vi "Encoder_sub_VI.vi"(8 "error in (no error)":errorcluster, 11 "Encoder Input":T2) -> (0 "error out":errorcluster, 3 "Encoder Output":T2)   [LabVIEW 2017]
uses:
  <vilib>/myRIO/Common/Instrument Driver Framework/myRIO v1.0/Encoder/typedefs/Encoder Count Direction Enum.ctl
  <vilib>/myRIO/Common/Instrument Driver Framework/myRIO v1.0/Encoder/typedefs/Encoder Signal Mode.ctl
  <vilib>/myRIO/Instrument Drivers/Onboard IO/Encoder/typedefs/Encoder Reference.ctl
  <vilib>/myRIO/Common/Instrument Driver Framework/Utilities/typedefs/myRIO Generic Hardware Reference.ctl
  <vilib>/myRIO/Common/Instrument Driver Framework/Utilities/typedefs/Hardware Version Enum.ctl
  <vilib>/myRIO/Common/Instrument Driver Framework/Utilities/typedefs/myRIO v1.0 Reference.ctl
  <vilib>/myRIO/Common/Instrument Driver Framework/Utilities/typedefs/Generic FPGA Reference.ctl
  <vilib>/myRIO/Common/Instrument Driver Framework/myRIO v1.0/Encoder/typedefs/Encoder Channels Enum.ctl
  <vilib>/myRIO/Common/Instrument Driver Framework/myRIO v1.0/Encoder/typedefs/Encoder Configuration v1.0.ctl
  <vilib>/userdefined/High Color/nirio_resource_hc.ctl
  <vilib>/myRIO/Common/Instrument Driver Framework/Utilities/vis/Is FPGA Ref Available.vi
  <vilib>/myRIO/Common/Instrument Driver Framework/myRIO v1.0/Encoder/vis/myRIO v1.1 Open Encoder.vi
  <vilib>/myRIO/Instrument Drivers/Onboard IO/Encoder/vis/Read.vi
  <vilib>/myRIO/Common/Instrument Driver Framework/Utilities/vis/Validate Channels.vi
  <vilib>/myRIO/Common/Instrument Driver Framework/myRIO v1.0/Encoder/vis/myRIO v1.0 Reserve Encoder.vi
  <vilib>/myRIO/Common/Instrument Driver Framework/myRIO v1.0/Encoder/vis/myRIO v1.0 Build MUX Configuration Encoder.vi
  <vilib>/myRIO/Common/Instrument Driver Framework/myRIO v1.0/Resource Manager/vis/myRIO v1.0 Reserve Channel List.vi
  <vilib>/myRIO/Common/Instrument Driver Framework/myRIO v1.0/Resource Manager/vis/myRIO v1.0 Create Configuration List.vi
  <vilib>/myRIO/Common/Instrument Driver Framework/myRIO v1.0/Resource Manager/vis/myRIO v1.0 Reserve Channel.vi
  <vilib>/myRIO/Common/Instrument Driver Framework/myRIO v1.0/Resource Manager/vis/myRIO v1.0 Unreserve Channel.vi
  <vilib>/myRIO/Common/Instrument Driver Framework/myRIO v1.0/Resource Manager/vis/myRIO v1.0 Build Mutex Name.vi
  <vilib>/Utility/VariantDataType/GetNumericInfo.vi
  <vilib>/Utility/error.llb/Error Cluster From Error Code.vi
  <vilib>/myRIO/Common/Instrument Driver Framework/myRIO v1.0/myRIO v1.1 Open.vi
  <vilib>/myRIO/Common/Instrument Driver Framework/Utilities/vis/IO Manager.vi
  <vilib>/myRIO/Common/Instrument Driver Framework/Utilities/vis/Configuration Manager.vi
  <vilib>/myRIO/Common/Instrument Driver Framework/myRIO v1.0/Resource Manager/vis/myRIO v1.0 Configure IO.vi
  <vilib>/myRIO/Common/Instrument Driver Framework/myRIO v1.0/myRIO v1.0 Close.vi
  <vilib>/myRIO/Common/Instrument Driver Framework/myRIO v1.0/Encoder/vis/myRIO v1.0 Configure Encoder.vi
  <vilib>/myRIO/Common/Instrument Driver Framework/myRIO v1.0/Encoder/vis/myRIO v1.0 Read Encoder.vi
  <vilib>/myRIO/Express VI/Onboard IO/Encoder/Encoder Express VI.xnode
  <vilib>/myRIO/Instrument Drivers/Onboard IO/Encoder/vis/myRIO Encoder Open.xnode
  <vilib>/myRIO/Instrument Drivers/Onboard IO/Encoder/Encoder.lvlib
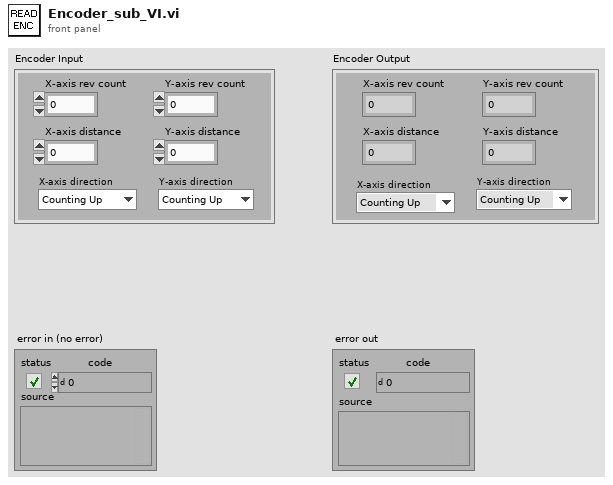
[diagram p1: front panel]
types:
  T1 = typedef "Encoder Count Direction Enum.ctl" = enum16{"Counting Up", "Counting Down"}
  T2 = cluster{"Y-axis rev count":dbl, "Y-axis distance":dbl, "X-axis rev count":dbl, "X-axis distance":dbl, "Y-axis direction":T1, "X-axis direction":T1}
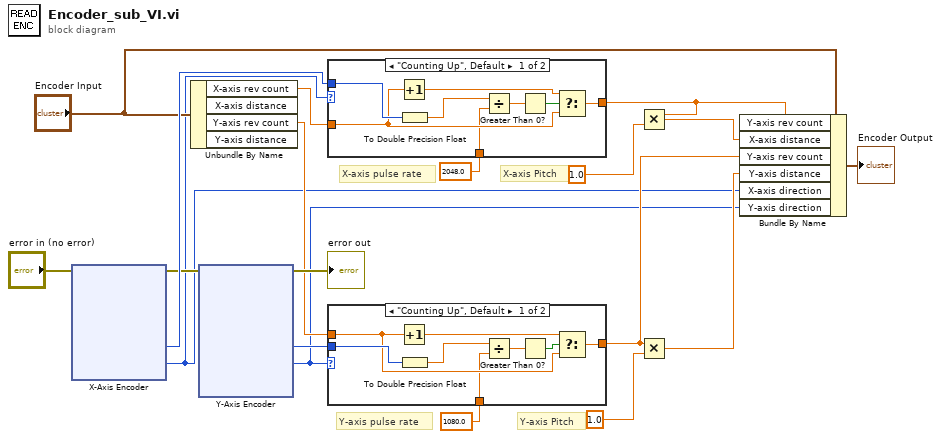
[diagram p0: block diagram]
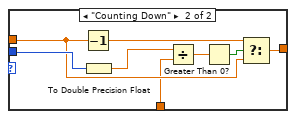
[diagram p2: hidden frame]
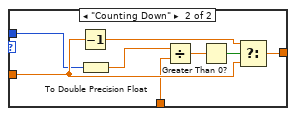
[diagram p3: hidden frame]
diagram:
  # "Y-axis pulse rate"
  # "X-axis pulse rate"
  # "Y-axis Pitch"
  # "X-axis Pitch"
  n1 = xnode "X-Axis Encoder"("error in (no error)"="error in (no error)") -> ("Counter Value"=w16:i32, "Counter Direction"=w2:T1, "error out"=w14:errorcluster)  [unwired: 1 in, 1 out]
  n2 = Unbundle By Name("Encoder Input") -> ("X-axis rev count"=w6:dbl, "Y-axis rev count"=w7:dbl)  [unwired: 2 out]
  n3 = xnode "Y-Axis Encoder"("error in (no error)"=w14) -> ("Counter Value"=w17:i32, "Counter Direction"=w1:T1, "error out"=→"error out":errorcluster)  [unwired: 1 in, 1 out]
  n4 = case shown="\"Counting Up\", Default" w2 {
    tunnel: w16 -> [w27 w30]
    tunnel: [w21 w29] -> w13
    tunnel: w6 -> [w22 w31]
    tunnel: 2048.0 -> [w20 w28]
    frame "Counting Up", Default {
      n5 = Increment(x=w22) -> (x+1=w23:dbl)
      n6 = To Double Precision Float(number=w27) -> (double precision float=w24:dbl)
      n7 = Divide(x=w24, y=w20) -> (x/y=w25:dbl)
      n8 = Greater Than 0?(x=w25) -> (x > 0?=w26:bool)
      n9 = Select(t=w23, s=w26, f=w22) -> (s? t:f=w21:dbl)
    }
    frame "Counting Down" {
      n10 = Decrement(x=w31) -> (x-1=w32:dbl)
      n11 = To Double Precision Float(number=w30) -> (double precision float=w33:dbl)
      n12 = Divide(x=w33, y=w28) -> (x/y=w34:dbl)
      n13 = Greater Than 0?(x=w34) -> (x > 0?=w35:bool)
      n14 = Select(t=w32, s=w35, f=w31) -> (s? t:f=w29:dbl)
    }
  }
  n15 = case shown="\"Counting Up\", Default" w1 {
    tunnel: w17 -> [w39 w46]
    tunnel: [w37 w47] -> w8
    tunnel: w7 -> [w38 w45]
    tunnel: 1080.0 -> [w36 w44]
    frame "Counting Up", Default {
      n16 = Increment(x=w38) -> (x+1=w40:dbl)
      n17 = To Double Precision Float(number=w39) -> (double precision float=w41:dbl)
      n18 = Divide(x=w41, y=w36) -> (x/y=w42:dbl)
      n19 = Greater Than 0?(x=w42) -> (x > 0?=w43:bool)
      n20 = Select(t=w40, s=w43, f=w38) -> (s? t:f=w37:dbl)
    }
    frame "Counting Down" {
      n21 = Decrement(x=w45) -> (x-1=w51:dbl)
      n22 = To Double Precision Float(number=w46) -> (double precision float=w50:dbl)
      n23 = Divide(x=w50, y=w44) -> (x/y=w49:dbl)
      n24 = Greater Than 0?(x=w49) -> (x > 0?=w48:bool)
      n25 = Select(t=w51, s=w48, f=w45) -> (s? t:f=w47:dbl)
    }
  }
  n26 = Multiply(x=w13, y=1.0) -> (x*y=w12:dbl)
  n27 = Multiply(x=w8, y=1.0) -> (x*y=w11:dbl)
  n28 = Bundle By Name(cluster="Encoder Input", "Y-axis rev count"=w13, "X-axis distance"=w12, "Y-axis rev count"=w8, "Y-axis distance"=w11, "X-axis direction"=w2, "Y-axis direction"=w1) -> (→"Encoder Output":T2)
